vi "test trigger.vi"() -> ()   [LabVIEW 2012]
uses:
  <vilib>/Instr/_visa.llb/VISA Configure Serial Port (Instr).vi
  <vilib>/DAQmx/write.llb/DAQmx Write (Analog 1D Wfm NChan NSamp).vi
  <vilib>/DAQmx/configure/timing.llb/DAQmx Timing (Sample Clock).vi
  <resource>/objmgr/daqmx.rc
  <vilib>/measure/NI_MABase.lvlib
  <vilib>/DAQmx/configure/trigger.llb/DAQmx Start Trigger (Digital Edge).vi
  <vilib>/DAQmx/configure/trigger.llb/DAQmx Start Trigger (Analog Edge).vi
  <vilib>/DAQmx/configure/trigger.llb/DAQmx Reference Trigger (Digital Edge).vi
  <vilib>/DAQmx/configure/trigger.llb/DAQmx Reference Trigger (Analog Edge).vi
  <vilib>/DAQmx/read.llb/DAQmx Read (Analog 1D Wfm NChan NSamp).vi
  <vilib>/DAQmx/configure/task.llb/DAQmx Configure Logging (TDMS).vi
  <vilib>/DAQmx/create/channels.llb/DAQmx Create Channel (AO-Voltage-Basic).vi
  <vilib>/DAQmx/create/channels.llb/DAQmx Create Channel (AI-Voltage-Basic).vi
panel:
  in  "Line Scan":bool
  out "Move X":bool
  in  "Step X":dbl=0.2
  in  "Emergency Stop":bool
  in  "Stop 3":bool
  in  "Home Y":bool
  in  "Home X":bool
  in  "Back":bool
  in  "Front":bool
  in  "Left":bool
  in  "Right":bool
  in  "Save Speed":bool
  in  "Stop Scan":bool
  in  "Cur. Pos Y":dbl=30.0 format="%#.4f"
  in  "Cur. Pos X":dbl=-33.28 format="%#.4f"
  in  "Travel per Pulse (mm)":dbl=0.002
  in  "2 Rate":dbl=0.4
  in  "1 Rate":dbl=0.2
  in  "Step Y":dbl=0.2
  in  "Y-length":dbl=20.0
  in  "X-length":dbl=20.0
  in  "2 Min":dbl=0.4
  in  "1  Max":dbl=6.0
  in  "2 Max":dbl=6.0
  in  "1 Min":dbl=0.4
  in  "Parity":u16(ring) items=["None", "Odd", "Even", "Mark", "Space"]
  in  "stop bits":u16(ring)=10 items=["1.0"=10, "1.5"=15, "2.0"=20]
  in  "Move Distance (mm)":dbl=10.0
  in  "Data bits":u16=8 min=5 max=8 step=1
  in  "Baud Rate":u32=9600
  in  "COM Port":refnum<visa-resource-name>="COM4"
  in  "Scan":bool
  out "Waveform Graph":waveform(dbl)[](graph)=[{"t0"=timestamp(3527210060.2234635 s since 1904-01-01), "dt"=1.9999999999999944e-06, "Y"=array[5000 elements], "attributes"=variant("NI_ChannelName"=variant(string "Dev4/ai1"), "NI_UnitDescription"=variant(string "Volts"))}]
  out "숫자형":i32=2
  in  "Number of Samples 2":i32=5000
  in  "Trigger Type":T1(tab)=enum."Digital Start"
  in  "Edge":i32(ring)=10280 items=["Rising"=10280, "Falling"=10171]
  in  "Digital Trigger Source":tag="/Dev4/PFI1"
  in  "Level (V)":dbl format="%0.2f"
  in  "Hysteresis (V)":dbl
  in  "Slope":i32(ring)=10280 items=["Rising"=10280, "Falling"=10171]
  in  "Analog Trigger Source":string="APFI0"
  in  "Digital Ref Trigger Source":tag
  in  "Edge 2":i32(ring)=10280 items=["Rising"=10280, "Falling"=10171]
  in  "Pre-Trigger Samples":u32
  in  "Analog Ref Trigger Source":string="APFI0"
  in  "Slope 2":i32(ring)=10280 items=["Rising"=10280, "Falling"=10171]
  in  "Level (V) 2":dbl format="%0.2f"
  in  "Pre-Trigger Samples 2":u32
  in  "TDMS File Path":path
  in  "Sample Rate":dbl=500000.0
  in  "Sample Clock Source 2":tag="OnboardClock"
  in  "Terminal Configuration":i32(ring)=10083 items=["default"=-1, "RSE"=10083, "NRSE"=10078, "Differential"=10106, "Pseudodifferential"=12529]
  in  "Max Voltage":dbl=10.0
  in  "Min Voltage":dbl=-10.0
  in  "Physical Channel":tag="Dev4/ai1"
  out "Actual Sample Rate":dbl=500000.0 format="%0.2f"
  in  "Logging Mode":i32(ring)=10231 items=["Off"=10231, "Log and Read"=15842]
  in  "Stop 4":bool
  out "Actual Sample Rate 2":dbl=500000.0 format="%0.2f"
  in  "Physical Channel(s)":tag="Dev4/ao1"
  in  "Min Voltage 2":dbl=-10.0
  in  "Max Voltage 2":dbl=10.0
  in  "Sample Clock Source":tag="OnboardClock"
  in  "Sample Rate 2":dbl=500000.0
  in  "Number of Samples":i32=6000
  in  "Output Array":T2(array[cluster])=[{"Waveform Type"=2, "Amplitude"=5.0, "Frequency"=2000.0}] {"Frequency" format="%0.2p"; "Amplitude" format="%0.2p"; "Waveform Type" items=["Sine Wave", "Triangle Wave", "Square Wave", "Sawtooth Wave"]}
  in  "Duty cycle %":dbl=50.0 format="%#.2f"
  in  "Pulser Trigger Source":tag="/Dev4/PFI1" caption="소스"
  out "Waveform Graph 2":waveform(dbl)[](graph)=[{"t0"=timestamp(0 s since 1904-01-01), "dt"=2e-06, "Y"=array[6000 elements]}]
  # "Motor"
  # "Measure Pulser"
  # "Pulser Out"
  # "To configure and use a start trigger you must have the necessary tab selected above.  Not all hardware supports triggering--refer to your device documentation for more info."
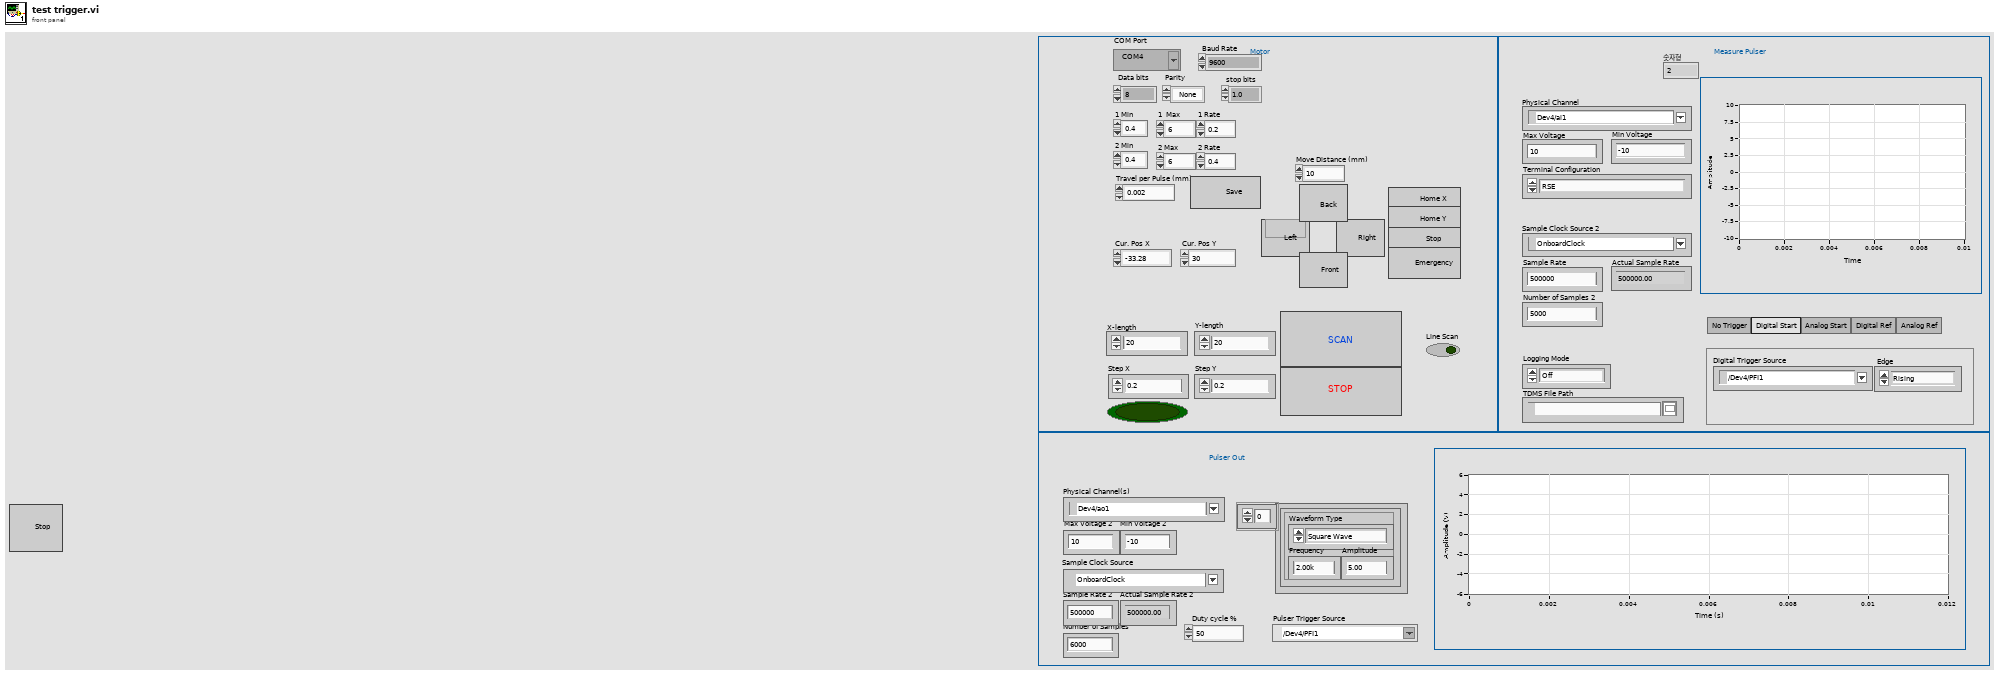
[diagram p1: front panel]
types:
  T1 = enum32{"No Trigger", "Digital Start", "Analog Start", "Digital Ref", "Analog Ref"}
  T2 = cluster{"Waveform Type":u16, "Amplitude":dbl, "Frequency":dbl}[]
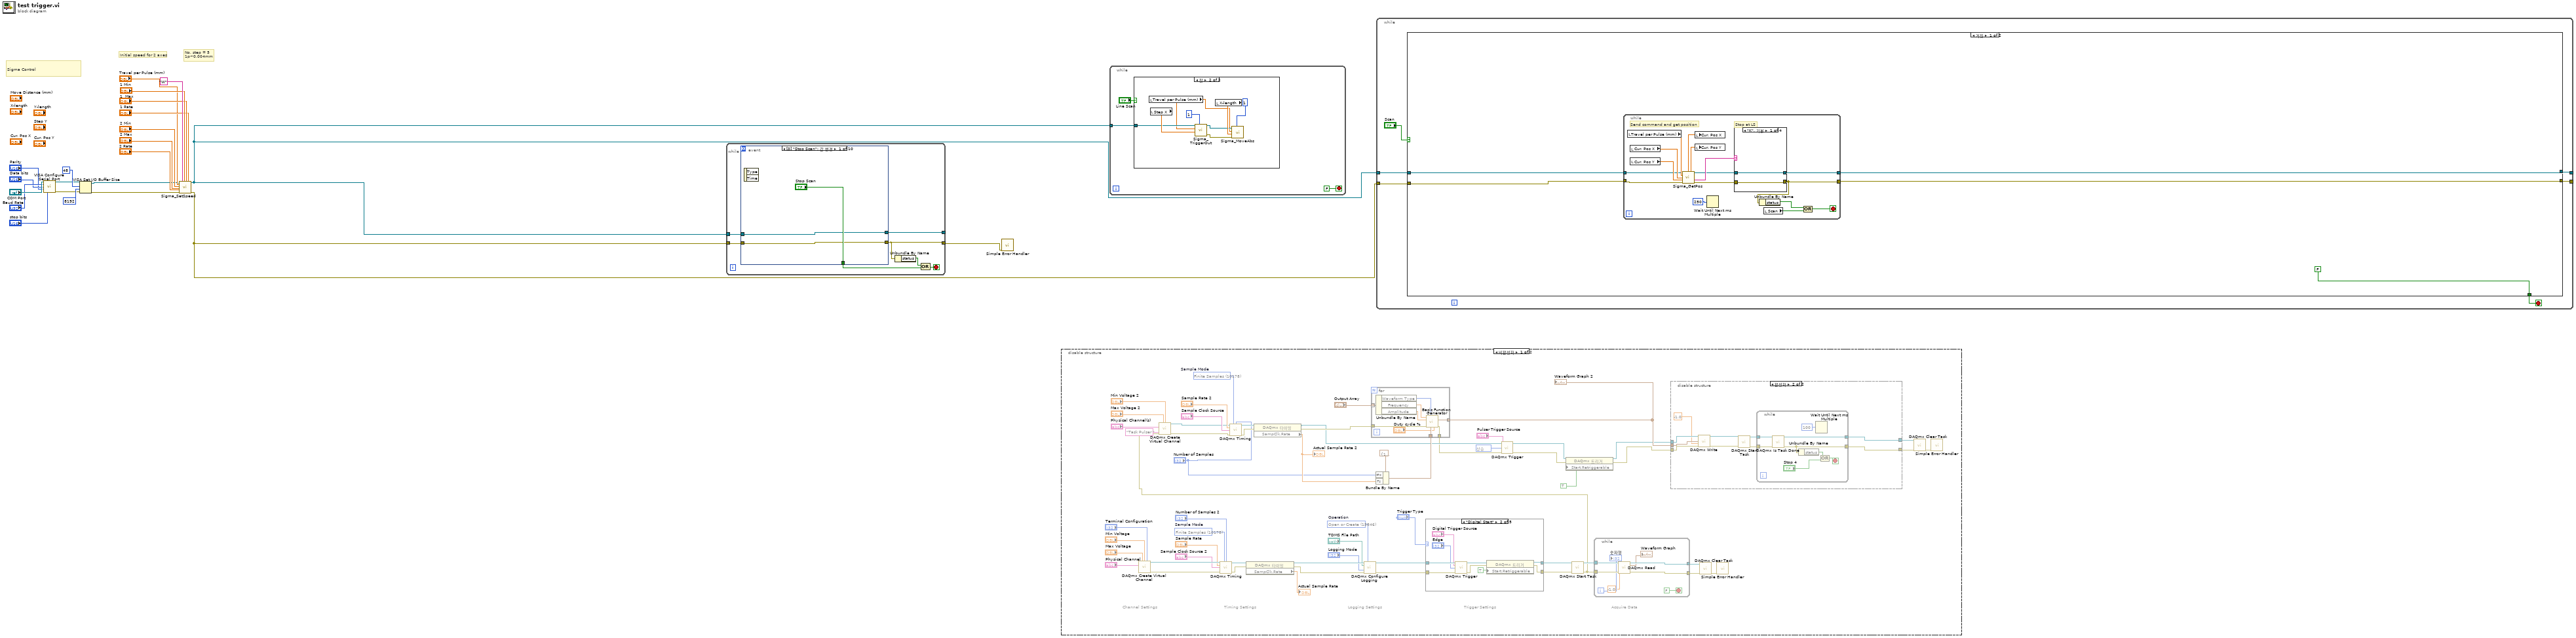
[diagram p0: block diagram]
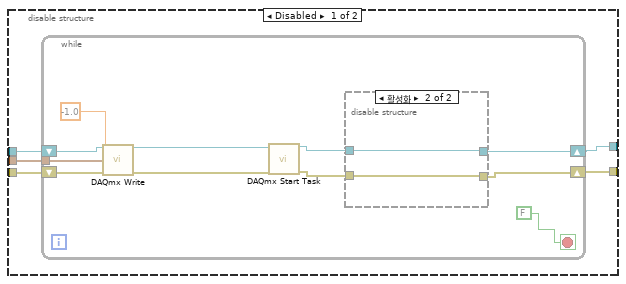
[diagram p2: hidden frame]
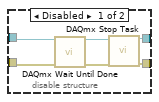
[diagram p3: hidden frame]
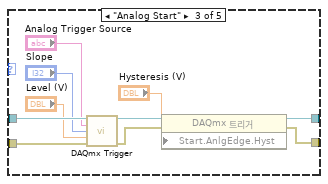
[diagram p5: hidden frame]
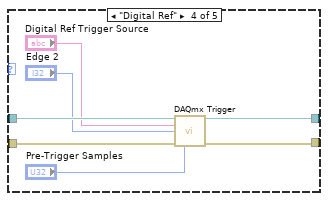
[diagram p6: hidden frame]
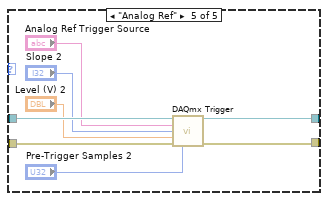
[diagram p7: hidden frame]
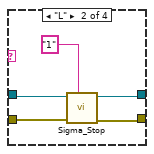
[diagram p10: hidden frame]
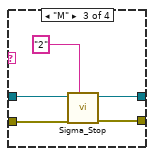
[diagram p11: hidden frame]
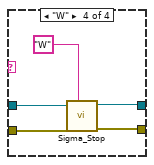
[diagram p12: hidden frame]
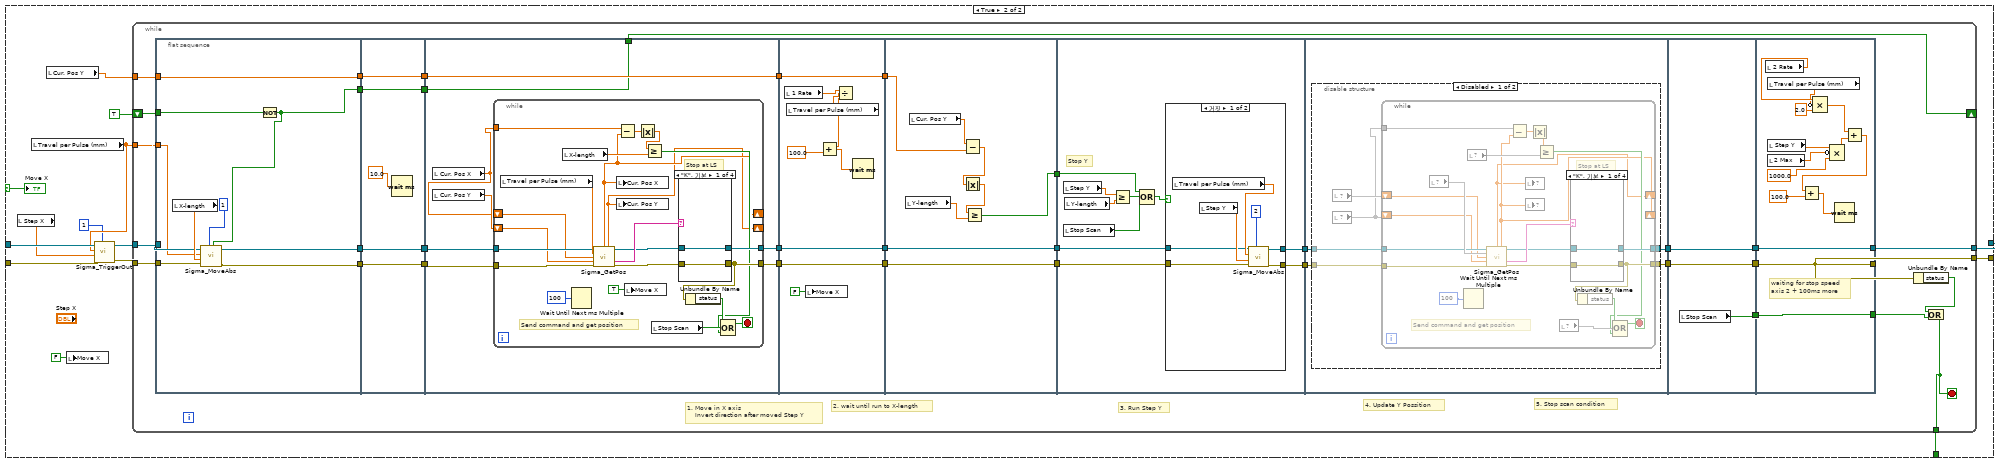
[diagram p13: hidden frame]
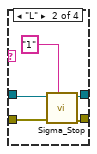
[diagram p14: hidden frame]
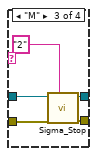
[diagram p15: hidden frame]
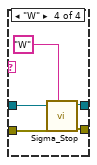
[diagram p16: hidden frame]
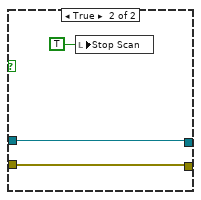
[diagram p17: hidden frame]
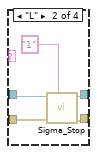
[diagram p18: hidden frame]
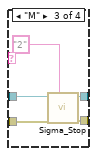
[diagram p19: hidden frame]
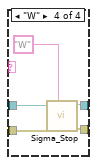
[diagram p20: hidden frame]
diagram:
  # "No. step = 5\n1p~0.004mm"
  # "Initial speed for 2 axes"
  # "Sigma Control"
  n1 = call-poly "VISA Configure Serial Port"("VISA resource name"="COM Port", "baud rate (9600)"="Baud Rate", "data bits (8)"="Data bits", "parity (0:none)"="Parity", "stop bits (10: 1 bit)"="stop bits") -> ("VISA resource name out"=w9:refnum<visa-resource-name>, "error out"=w3:errorcluster)  [unwired: 9 in]
  n2 = VISA Set I/O Buffer Size(VISA resource name=w9, mask (16)=48, size (4096)=u32 8192, error in (no error)=w3) -> (VISA resource name out=w13:refnum<visa-resource-name>, error out=w12:errorcluster)
  n3 = call "Sigma_SetSpeed.vi"("VISA resource name"=w13, "Travel per Pulse (0.004mm)"="Travel per Pulse (mm)", "Min (1mm) 2"="2 Min", "Max (2mm) 2"="2 Max", "Rate (1mm) 2"="2 Rate", "error in (no error)"=w12, "Axis (1)"="W", "Min (1mm)"="1 Min", "Max (2mm)"="1  Max", "Rate (1mm)"="1 Rate") -> ("VISA resource name out"=w1:refnum<visa-resource-name>, "error out"=w2:errorcluster)  [unwired: 8 in]
  n4 = while {
    tunnel: w1 -> [w29]
    tunnel: [w24] -> _
    tunnel: w2 -> [w28]
    tunnel: [w26] -> w22
    stop <- w25 stop-if-true
    n5 = event shown="[0] \"Stop Scan\": 값 변경" {
      selector: _ -> [_ _ _ _ _ _ _ _ _ _]
      dyn-events: _ -> [_ _ _ _ _ _ _ _ _ _]
      timeout: _ -> [_ _ _ _ _ _ _ _ _ _]
      tunnel: w29 -> [w31 w44 w47 w62 w77 w92 w109 w121 w131 w143]
      tunnel: w28 -> [w30 w41 w46 w61 w76 w91 w108 w120 w130 w142]
      tunnel: [w31 w43 w49 w64 w79 w94 w106 w119 w133 w145] -> w24
      tunnel: [w30 w42 w48 w63 w78 w93 w105 w118 w132 w144] -> w26
      tunnel: ["Stop Scan" _ _ _ _ _ _ _ _ _] -> w23
      event "Stop Scan": Value Change {
        n6 = event-data() -> ()  [unwired: 1 in, 2 out]
      }
      event "Save Speed": Value Change {
        n7 = event-data() -> ()  [unwired: 1 in, 5 out]
        n8 = local read "Travel per Pulse (mm)"() -> (w33:dbl)
        n9 = local read "1  Max"() -> (w38:dbl)
        n10 = local read "1 Rate"() -> (w37:dbl)
        n11 = local read "2 Rate"() -> (w34:dbl)
        n12 = local read "2 Max"() -> (w35:dbl)
        n13 = local read "1 Min"() -> (w39:dbl)
        n14 = local read "2 Min"() -> (w36:dbl)
        n15 = call "Sigma_SetSpeed.vi"("VISA resource name"=w44, "Travel per Pulse (0.004mm)"=w33, "Min (1mm) 2"=w36, "Max (2mm) 2"=w35, "Rate (1mm) 2"=w34, "error in (no error)"=w41, "Axis (1)"="W", "Min (1mm)"=w39, "Max (2mm)"=w38, "Rate (1mm)"=w37) -> ("VISA resource name out"=w43:refnum<visa-resource-name>, "error out"=w42:errorcluster)  [unwired: 8 in]
      }
      event "Right": Value Change {
        n16 = event-data() -> ()  [unwired: 1 in, 1 out]
        n17 = case shown="참" "Right" {
          tunnel: [w51 w57] -> w49
          tunnel: [w50 w56] -> w48
          tunnel: w47 -> [w51 w59]
          tunnel: w46 -> [w50 w58]
          frame False {
          }
          frame True {
            n18 = local read "Travel per Pulse (mm)"() -> (w53:dbl)
            n19 = local read "Move Distance (mm)"() -> (w52:dbl)
            n20 = call "Sigma_MoveAbs.vi"("Direction (+)"=FALSE, "Axis (1)"=1, "error in (no error)"=w58, "Travel (1mm)"=w52, "Travel per Pulse (0.004mm)"=w53, "VISA resource name"=w59) -> ("error out"=w56:errorcluster, "VISA resource name out"=w57:refnum<visa-resource-name>)  [unwired: 4 in]
          }
        }
      }
      event "Left": Value Change {
        n21 = event-data() -> ()  [unwired: 1 in, 1 out]
        n22 = case shown="참" "Left" {
          tunnel: [w66 w73] -> w64
          tunnel: [w65 w72] -> w63
          tunnel: w62 -> [w66 w74]
          tunnel: w61 -> [w65 w71]
          frame False {
          }
          frame True {
            n23 = local read "Travel per Pulse (mm)"() -> (w68:dbl)
            n24 = local read "Move Distance (mm)"() -> (w67:dbl)
            n25 = call "Sigma_MoveAbs.vi"("Direction (+)"=TRUE, "Axis (1)"=1, "error in (no error)"=w71, "Travel (1mm)"=w67, "Travel per Pulse (0.004mm)"=w68, "VISA resource name"=w74) -> ("error out"=w72:errorcluster, "VISA resource name out"=w73:refnum<visa-resource-name>)  [unwired: 4 in]
          }
        }
      }
      event "Front": Value Change {
        n26 = event-data() -> ()  [unwired: 1 in, 1 out]
        n27 = case shown="참" "Front" {
          tunnel: [w81 w87] -> w79
          tunnel: [w80 w86] -> w78
          tunnel: w77 -> [w81 w89]
          tunnel: w76 -> [w80 w88]
          frame False {
          }
          frame True {
            n28 = local read "Travel per Pulse (mm)"() -> (w83:dbl)
            n29 = local read "Move Distance (mm)"() -> (w82:dbl)
            n30 = call "Sigma_MoveAbs.vi"("Direction (+)"=FALSE, "Axis (1)"=2, "error in (no error)"=w88, "Travel (1mm)"=w82, "Travel per Pulse (0.004mm)"=w83, "VISA resource name"=w89) -> ("error out"=w86:errorcluster, "VISA resource name out"=w87:refnum<visa-resource-name>)  [unwired: 4 in]
          }
        }
      }
      event "Back": Value Change {
        n31 = event-data() -> ()  [unwired: 1 in, 1 out]
        n32 = case shown="참" "Back" {
          tunnel: [w96 w102] -> w94
          tunnel: [w95 w101] -> w93
          tunnel: w92 -> [w96 w104]
          tunnel: w91 -> [w95 w103]
          frame False {
          }
          frame True {
            n33 = local read "Travel per Pulse (mm)"() -> (w98:dbl)
            n34 = local read "Move Distance (mm)"() -> (w97:dbl)
            n35 = call "Sigma_MoveAbs.vi"("Direction (+)"=TRUE, "Axis (1)"=2, "error in (no error)"=w103, "Travel (1mm)"=w97, "Travel per Pulse (0.004mm)"=w98, "VISA resource name"=w104) -> ("error out"=w101:errorcluster, "VISA resource name out"=w102:refnum<visa-resource-name>)  [unwired: 4 in]
          }
        }
      }
      event "Home X": Value Change {
        n36 = event-data() -> ()  [unwired: 1 in, 1 out]
        n37 = case shown="참" "Home X" {
          tunnel: [w111 w114] -> w106
          tunnel: [w110 w113] -> w105
          tunnel: w109 -> [w111 w116]
          tunnel: w108 -> [w110 w115]
          frame False {
          }
          frame True {
            n38 = call "Sigma_Home.vi"("Axis (1)"="1", "error in (no error)"=w115, "VISA resource name"=w116) -> ("error out"=w113:errorcluster, "VISA resource name out"=w114:refnum<visa-resource-name>)  [unwired: 7 in]
          }
        }
      }
      event "Home Y": Value Change {
        n39 = event-data() -> ()  [unwired: 1 in, 1 out]
        n40 = case shown="참" "Home Y" {
          tunnel: [w123 w126] -> w119
          tunnel: [w122 w125] -> w118
          tunnel: w121 -> [w123 w128]
          tunnel: w120 -> [w122 w127]
          frame False {
          }
          frame True {
            n41 = call "Sigma_Home.vi"("Axis (1)"="2", "error in (no error)"=w127, "VISA resource name"=w128) -> ("error out"=w125:errorcluster, "VISA resource name out"=w126:refnum<visa-resource-name>)  [unwired: 7 in]
          }
        }
      }
      event "Stop 3": Value Change {
        n42 = event-data() -> ()  [unwired: 1 in, 1 out]
        n43 = case shown="참" "Stop 3" {
          tunnel: [w135 w136] -> w133
          tunnel: [w134 w137] -> w132
          tunnel: w131 -> [w135 w139]
          tunnel: w130 -> [w134 w138]
          frame False {
          }
          frame True {
            n44 = call "Sigma_Stop.vi"("Axis (1)"="W", "error in (no error)"=w138, "VISA resource name"=w139) -> ("error out"=w137:errorcluster, "VISA resource name out"=w136:refnum<visa-resource-name>)  [unwired: 7 in]
          }
        }
      }
      event "Emergency Stop": Value Change {
        n45 = event-data() -> ()  [unwired: 1 in, 1 out]
        n46 = case shown="참" "Emergency Stop" {
          tunnel: [w147 w150] -> w145
          tunnel: [w146 w149] -> w144
          tunnel: w143 -> [w147 w152]
          tunnel: w142 -> [w146 w151]
          frame False {
          }
          frame True {
            n47 = call "Sigma_Stop.vi"("Axis (1)"="E", "error in (no error)"=w151, "VISA resource name"=w152) -> ("error out"=w149:errorcluster, "VISA resource name out"=w150:refnum<visa-resource-name>)  [unwired: 7 in]
          }
        }
      }
    }
    n48 = Unbundle By Name(w26) -> ("status"=w27:bool)
    n49 = Compound Arithmetic op=OR(w27, w23) -> (w25:bool)
  }
  n50 = call <vilib>:"Simple Error Handler.vi"("error in (no error)"=w22) -> ()  [unwired: 4 in, 5 out]
  n51 = disable-structure shown="비활성화" {
    frame Disabled {
      w165 = 10280 items=["상승"=10280, "하강"=10171] ("edge")
      w181 = 10178 items=["Finite Samples"=10178, "Continuous Samples"=10123, "Hardware Timed Single Point"=12522]  # Sample Mode
      w203 = 15846 items=["Open"=10437, "Open or Create"=15846, "Create or Replace"=15847, "Create"=15848]  # Operation
      w208 = 10178 items=["Finite Samples"=10178, "Continuous Samples"=10123, "Hardware Timed Single Point"=12522]  # Sample Mode
      # "Acquire Data"
      # "Trigger Settings"
      # "Timing Settings"
      # "Channel Settings"
      # "Logging Settings"
      n52 = call-poly <vilib>:"DAQmx Create Virtual Channel.vi"("maximum value"="Max Voltage", "minimum value"="Min Voltage", "input terminal configuration"="Terminal Configuration", "physical channels"="Physical Channel") -> ("task out"=w206:refnum<k21>, "error out"=w207:errorcluster)  [unwired: 10 in]
      n53 = call-poly <vilib>:"DAQmx Timing.vi"("task/channels in"=w206, "sample mode"=w208, "samples per channel"="Number of Samples 2", "rate"="Sample Rate", "source"="Sample Clock Source 2", "error in"=w207) -> ("task out"=w210:refnum<k21>, "error out"=w209:errorcluster)  [unwired: 8 in]
      n54 = property class="DAQmx 타이밍"(reference=w210, error in=w209) -> (reference out=w205:refnum<k21>, error out=w204:errorcluster, "SampClk.Rate"=→"Actual Sample Rate":dbl)
      n55 = call-poly <vilib>:"DAQmx Configure Logging.vi"("task/channels in"=w205, "operation"=w203, "file path"="TDMS File Path", "logging mode"="Logging Mode", "error in"=w204) -> ("task out"=w202:refnum<k21>, "error out"=w201:errorcluster)  [unwired: 9 in]
      n56 = case shown="\"Digital Start\"" "Trigger Type" {
        tunnel: w202 -> [w271 w280 w290 w297 w305]
        tunnel: w201 -> [w270 w279 w289 w296 w304]
        tunnel: [w271 w275 w287 w295 w299] -> w200
        tunnel: [w270 w274 w286 w294 w300] -> w199
        frame "No Trigger", Default {
        }
        frame "Digital Start" {
          n57 = call-poly <vilib>:"DAQmx Trigger.vi"("task/channels in"=w280, "source"="Digital Trigger Source", "edge"="Edge", "error in"=w279) -> ("task out"=w276:refnum<k21>, "error out"=w273:errorcluster)  [unwired: 10 in]
          n58 = property class="DAQmx 트리거"(reference=w276, error in=w273, "Start.Retriggerable"=TRUE ("시작:추가 옵션:재트리거 가능")) -> (reference out=w275:refnum<k21>, error out=w274:errorcluster)
        }
        frame "Analog Start" {
          n59 = call-poly <vilib>:"DAQmx Trigger.vi"("task/channels in"=w290, "source"="Analog Trigger Source", "slope"="Slope", "level"="Level (V)", "error in"=w289) -> ("task out"=w285:refnum<k21>, "error out"=w284:errorcluster)  [unwired: 9 in]
          n60 = property class="DAQmx 트리거"(reference=w285, error in=w284, "Start.AnlgEdge.Hyst"="Hysteresis (V)") -> (reference out=w287:refnum<k21>, error out=w286:errorcluster)
        }
        frame "Digital Ref" {
          n61 = call-poly <vilib>:"DAQmx Trigger.vi"("task/channels in"=w297, "source"="Digital Ref Trigger Source", "edge"="Edge 2", "error in"=w296, "pretrigger samples per channel"="Pre-Trigger Samples") -> ("task out"=w295:refnum<k21>, "error out"=w294:errorcluster)  [unwired: 9 in]
        }
        frame "Analog Ref" {
          n62 = call-poly <vilib>:"DAQmx Trigger.vi"("task/channels in"=w305, "source"="Analog Ref Trigger Source", "slope"="Slope 2", "level"="Level (V) 2", "error in"=w304, "pretrigger samples per channel"="Pre-Trigger Samples 2") -> ("task out"=w299:refnum<k21>, "error out"=w300:errorcluster)  [unwired: 8 in]
        }
      }
      n63 = call <vilib>:"DAQmx Start Task.vi"("task/channels in"=w200, "error in"=w199) -> ("task out"=w198:refnum<k21>, "error out"=w154:errorcluster)  [unwired: 12 in]
      n64 = call-poly <vilib>:"DAQmx Create Virtual Channel.vi"("maximum value"="Max Voltage 2", "minimum value"="Min Voltage 2", "physical channels"="Physical Channel(s)", "name to assign"="Task Pulser ", "error in"=w154) -> ("task out"=w163:refnum<k21>, "error out"=w162:errorcluster)  [unwired: 9 in]
      n65 = call-poly <vilib>:"DAQmx Timing.vi"("task/channels in"=w163, "sample mode"=w181, "samples per channel"="Number of Samples", "rate"="Sample Rate 2", "source"="Sample Clock Source", "error in"=w162) -> ("task out"=w183:refnum<k21>, "error out"=w182:errorcluster)  [unwired: 8 in]
      n66 = property class="DAQmx 타이밍"(reference=w183, error in=w182) -> (reference out=w168:refnum<k21>, error out=w174:errorcluster, "SampClk.Rate"=w172:dbl)
      "Actual Sample Rate 2" <- w172
      n67 = Bundle By Name(cluster=cluster{"Fs":dbl, "#s":dbl} {"Fs"=1000.0, "#s"=1000.0} ("sampling info"), "#s"="Number of Samples", "Fs"=w172) -> (w171:cluster{"Fs":dbl, "#s":dbl})
      n68 = for {
        tunnel: w174 -> [w219]
        tunnel: w171 -> [w218]
        tunnel: [w217] -> w167
        tunnel: "Output Array" -> [w216] mode=indexing
        tunnel: [w213] -> w170 mode=indexing
        n69 = Unbundle By Name(w216) -> ("Waveform Type"=w215:u16, "Frequency"=w214:dbl, "Amplitude"=w211:dbl)
        n70 = call <vilib>:"Basic Function Generator.vi"("square wave duty cycle (%)"="Duty cycle %", "sampling info"=w218, "signal type"=w215, "error in (no error)"=w219, "amplitude"=w211, "frequency"=w214) -> ("error out"=w217:errorcluster, "signal out"=w213:waveform(dbl))  [unwired: 3 in, 1 out]
      }
      "Waveform Graph 2" <- w170
      n71 = call-poly <vilib>:"DAQmx Trigger.vi"("task/channels in"=w168, "source"="Pulser Trigger Source", "edge"=w165, "error in"=w167) -> ("task out"=w159:refnum<k21>, "error out"=w155:errorcluster)  [unwired: 10 in]
      n72 = property class="DAQmx 트리거"(reference=w159, error in=w155, "Start.Retriggerable"=TRUE) -> (reference out=w158:refnum<k21>, error out=w157:errorcluster)
      n73 = while {
        tunnel: w198 -> [w269]
        tunnel: w154 -> [w268]
        tunnel: [w267] -> w197
        tunnel: [w266] -> w196
        i -> [w264]
        stop <- FALSE stop-if-true
        n74 = call-poly <vilib>:"DAQmx Read.vi"("task/channels in"=w269, "timeout"=-1.0, "error in"=w268) -> ("task out"=w267:refnum<k21>, "data"=→"Waveform Graph":waveform(dbl)[], "error out"=w266:errorcluster)  [unwired: 10 in]
        "숫자형" <- w264
      }
      n75 = disable-structure shown="활성화" {
        disable-tunnel: w170 -> [w224 w247]
        disable-tunnel: [w223 w246] -> w161
        disable-tunnel: [w222 w245] -> w160
        disable-tunnel: w158 -> [w221 w249]
        disable-tunnel: w157 -> [w220 w248]
        frame Disabled {
          n76 = while {
            tunnel: w224 -> [w235]
            shift-right: [w231] -> w223
            shift-left: w221 -> [w229]
            shift-right: [w230] -> w222
            shift-left: w220 -> [w228]
            stop <- FALSE stop-if-true
            n77 = call-poly <vilib>:"DAQmx Write.vi"("task/channels in"=w229, "data"=w235, "timeout"=-1.0, "error in"=w228) -> ("task out"=w234:refnum<k21>, "error out"=w233:errorcluster)  [unwired: 9 in, 1 out]
            n78 = call <vilib>:"DAQmx Start Task.vi"("task/channels in"=w234, "error in"=w233) -> ("task out"=w227:refnum<k21>, "error out"=w226:errorcluster)  [unwired: 12 in]
            n79 = disable-structure shown="활성화" {
              disable-tunnel: [w241 w243] -> w231
              disable-tunnel: [w240 w242] -> w230
              disable-tunnel: w227 -> [w239 w243]
              disable-tunnel: w226 -> [w238 w242]
              frame Disabled {
                n80 = call <vilib>:"DAQmx Wait Until Done.vi"("task/channels in"=w239, "error in"=w238) -> ("task out"=w237:refnum<k21>, "error out"=w236:errorcluster)  [unwired: 12 in]
                n81 = call <vilib>:"DAQmx Stop Task.vi"("task/channels in"=w237, "error in"=w236) -> ("task out"=w241:refnum<k21>, "error out"=w240:errorcluster)  [unwired: 12 in]
              }
              frame Enabled {
              }
            }
          }
        }
        frame Enabled {
          n82 = call-poly <vilib>:"DAQmx Write.vi"("task/channels in"=w249, "data"=w247, "timeout"=-1.0, "error in"=w248) -> ("task out"=w251:refnum<k21>, "error out"=w253:errorcluster)  [unwired: 9 in, 1 out]
          n83 = call <vilib>:"DAQmx Start Task.vi"("task/channels in"=w251, "error in"=w253) -> ("task out"=w250:refnum<k21>, "error out"=w252:errorcluster)  [unwired: 12 in]
          n84 = while {
            tunnel: w250 -> [w261]
            tunnel: w252 -> [w260]
            tunnel: [w258] -> w245
            tunnel: [w259] -> w246
            stop <- w254 stop-if-true
            n85 = call <vilib>:"DAQmx Is Task Done.vi"("task/channels in"=w261, "error in"=w260) -> ("task out"=w259:refnum<k21>, "error out"=w258:errorcluster)  [unwired: 11 in, 1 out]
            n86 = Unbundle By Name(w258) -> ("status"=w255:bool)
            n87 = Wait Until Next ms Multiple(millisecond multiple=u32 100) -> ()  [unwired: 1 out]
            n88 = Compound Arithmetic op=OR(w255, "Stop 4") -> (w254:bool)
          }
        }
      }
      n89 = call <vilib>:"DAQmx Clear Task.vi"("task in"=w197, "error in"=w196) -> ("error out"=w195:errorcluster)  [unwired: 13 in]
      n90 = call <vilib>:"Simple Error Handler.vi"("error in (no error)"=w195) -> ()  [unwired: 4 in, 5 out]
      n91 = call <vilib>:"DAQmx Clear Task.vi"("task in"=w161, "error in"=w160) -> ("error out"=w180:errorcluster)  [unwired: 13 in]
      n92 = call <vilib>:"Simple Error Handler.vi"("error in (no error)"=w180) -> ()  [unwired: 4 in, 5 out]
    }
    frame Enabled {
    }
  }
  n93 = while {
    tunnel: w1 -> [w308]
    stop <- FALSE stop-if-true
    n94 = case shown="참" "Line Scan" {
      tunnel: w308 -> [_ w310]
      frame False {
      }
      frame True {
        n95 = local read "Travel per Pulse (mm)"() -> (w309:dbl)
        n96 = local read "Step X"() -> (w315:dbl)
        n97 = call "Sigma_TriggerOut.vi"("Axis(1)"=1, "Trigger distance (mm)"=w315, "Travel per Pulse (mm)"=w309, "VISA resource name"=w310) -> ("error out"=w311:errorcluster, "VISA resource name out"=w312:refnum<visa-resource-name>)  [unwired: 6 in]
        n98 = local read "X-length"() -> (w313:dbl)
        n99 = call "Sigma_MoveAbs.vi"("Axis (1)"=1, "error in (no error)"=w311, "Travel (1mm)"=w313, "Travel per Pulse (0.004mm)"=w309, "VISA resource name"=w312) -> ()  [unwired: 5 in, 2 out]
      }
    }
  }
  n100 = while {
    tunnel: w1 -> [w322]
    tunnel: [w320] -> _
    tunnel: w2 -> [w321]
    tunnel: [w319] -> _
    stop <- w318 stop-if-true
    n101 = case shown="거짓" "Scan" {
      selector: "Scan" -> [_ w369]
      tunnel: [w324 w371] -> w320
      tunnel: w322 -> [w326 w368]
      tunnel: w321 -> [w325 w365]
      tunnel: [w323 w370] -> w319
      tunnel: [FALSE w373] -> w318
      frame False {
        n102 = while {
          tunnel: w325 -> [w335]
          tunnel: [w330] -> w324
          tunnel: [w329] -> w323
          tunnel: w326 -> [w328]
          stop <- w342 stop-if-true
          # "Stop at LS"
          # "Send command and get position"
          n103 = local read "Travel per Pulse (mm)"() -> (w338:dbl)
          n104 = local read "Cur. Pos X"() -> (w332:dbl)
          n105 = local read "Cur. Pos Y"() -> (w331:dbl)
          n106 = call "Sigma_GetPos.vi"("VISA resource name"=w328, "Travel per Pulse (mm)"=w338, "Init Pos X (mm)"=w332, "Init  Pos Y (mm)"=w331, "error in (no error)"=w335) -> ("Pos X (mm)"=w334:dbl, "Pos Y (mm)"=w333:dbl, "VISA resource name out"=w337:refnum<visa-resource-name>, "State String"=w339:string, "error out"=w336:errorcluster)  [unwired: 6 in]
          n107 = local write "Cur. Pos X"(w334) -> ()
          n108 = local write "Cur. Pos Y"(w333) -> ()
          n109 = Wait Until Next ms Multiple(millisecond multiple=u32 250) -> ()  [unwired: 1 out]
          n110 = case shown="\"K\", 기본" w339 {
            tunnel: [w345 w350 w355 w360] -> w330
            tunnel: [w344 w349 w354 w359] -> w329
            tunnel: w337 -> [w345 w347 w352 w357]
            tunnel: w336 -> [w344 w346 w351 w356]
            frame "K", Default {
            }
            frame "L" {
              n111 = call "Sigma_Stop.vi"("Axis (1)"="1", "error in (no error)"=w346, "VISA resource name"=w347) -> ("error out"=w349:errorcluster, "VISA resource name out"=w350:refnum<visa-resource-name>)  [unwired: 7 in]
            }
            frame "M" {
              n112 = call "Sigma_Stop.vi"("Axis (1)"="2", "error in (no error)"=w351, "VISA resource name"=w352) -> ("error out"=w354:errorcluster, "VISA resource name out"=w355:refnum<visa-resource-name>)  [unwired: 7 in]
            }
            frame "W" {
              n113 = call "Sigma_Stop.vi"("Axis (1)"="W", "error in (no error)"=w356, "VISA resource name"=w357) -> ("error out"=w359:errorcluster, "VISA resource name out"=w360:refnum<visa-resource-name>)  [unwired: 7 in]
            }
          }
          n114 = Unbundle By Name(w329) -> ("status"=w343:bool)
          n115 = local read "Scan"() -> (w341:bool)
          n116 = Compound Arithmetic op=OR(w343, w341) -> (w342:bool)
        }
      }
      frame True {
        n117 = local read "Step X"() -> (w364:dbl)
        n118 = local read "Travel per Pulse (mm)"() -> (w363:dbl)
        n119 = local read "Cur. Pos Y"() -> (w374:dbl)
        n120 = local write "Move X"(FALSE ("Move X")) -> ()
        n121 = call "Sigma_TriggerOut.vi"("Axis(1)"=1, "error in (no error)"=w365, "Trigger distance (mm)"=w364, "Travel per Pulse (mm)"=w363, "VISA resource name"=w368) -> ("error out"=w366:errorcluster, "VISA resource name out"=w367:refnum<visa-resource-name>)  [unwired: 5 in]
        n122 = while {
          shift-right: [w394] -> _
          shift-left: TRUE ("Direction (+)") -> [w407]
          tunnel: w374 -> [w406]
          tunnel: [w402] -> w373
          tunnel: w367 -> [w409]
          tunnel: w366 -> [w408]
          tunnel: [w395] -> w371
          tunnel: [w392] -> w370
          tunnel: w363 -> [w383]
          stop <- w402 stop-if-true
          # "5. Stop scan condition"
          # "3. Run Step Y"
          # "2. wait until run to X-length"
          # "1. Move in X axis\n    Invert direction after moved Step Y"
          # "4. Update Y Possition"
          n123 = flat-sequence {
            tunnel: w409 -> [w414]
            tunnel: w408 -> [w413]
            tunnel: w407 -> [w419]
            tunnel: w406 -> [w417]
            tunnel: [w418] -> w382
            tunnel: [w412] -> w380
            tunnel: [w411] -> w378
            tunnel: [w417] -> w376
            tunnel: w383 -> [w410]
            tunnel: w382 -> [w424]
            tunnel: [w424] -> w381
            tunnel: w380 -> [w423]
            tunnel: [w423] -> w379
            tunnel: w378 -> [w422]
            tunnel: [w422] -> w377
            tunnel: w376 -> [w421]
            tunnel: [w421] -> w375
            tunnel: w381 -> [w427]
            tunnel: w379 -> [w432]
            tunnel: w377 -> [w431]
            tunnel: w375 -> [w428]
            tunnel: [w430] -> w401
            tunnel: [w429] -> w400
            tunnel: [w428] -> w396
            tunnel: [w427] -> w394
            tunnel: [w480] -> w391
            tunnel: w401 -> [w480]
            tunnel: [w479] -> w389
            tunnel: w400 -> [w479]
            tunnel: [w478] -> w387
            tunnel: w396 -> [w478]
            tunnel: w391 -> [w488]
            tunnel: [w488] -> w390
            tunnel: w389 -> [w487]
            tunnel: [w487] -> w388
            tunnel: w387 -> [w482]
            tunnel: [w483] -> w386
            tunnel: [w498] -> w405
            tunnel: [w497] -> w404
            tunnel: w390 -> [w494]
            tunnel: w388 -> [w493]
            tunnel: w386 -> [w490]
            tunnel: w405 -> [w512]
            tunnel: w404 -> [w511]
            tunnel: [w510] -> w397
            tunnel: [w509] -> w393
            tunnel: [w561] -> w399
            tunnel: [w560] -> w398
            tunnel: w397 -> [w560]
            tunnel: w393 -> [w561]
            tunnel: [w559] -> w384
            tunnel: w399 -> [w574]
            tunnel: [w575] -> w392
            tunnel: w398 -> [w575]
            tunnel: [w574] -> w395
            tunnel: [w573] -> w385
            tunnel: w384 -> [w573]
            frame #0 {
              n124 = local read "X-length"() -> (w416:dbl)
              n125 = Not(x=w419) -> (.not. x?=w418:bool)
              n126 = call "Sigma_MoveAbs.vi"("Direction (+)"=w418, "Axis (1)"=1, "error in (no error)"=w413, "Travel (1mm)"=w416, "Travel per Pulse (0.004mm)"=w410, "VISA resource name"=w414) -> ("error out"=w411:errorcluster, "VISA resource name out"=w412:refnum<visa-resource-name>)  [unwired: 4 in]
            }
            frame #1 {
              n127 = Wait (ms)(milliseconds to wait=10.0 ("y")) -> ()  [unwired: 1 out]
            }
            frame #2 {
              n128 = local read "Cur. Pos X"() -> (w425:dbl)
              n129 = local read "Cur. Pos Y"() -> (w426:dbl)
              n130 = while {
                tunnel: w432 -> [w445]
                tunnel: w431 -> [w446]
                tunnel: [w444] -> w430
                tunnel: [w443] -> w429
                shift-right: [w437] -> _
                shift-left: w426 -> [w436]
                shift-right: [w438] -> _
                shift-left: w425 -> [w435]
                tunnel: w425 -> [w434]
                stop <- w453 stop-if-true
                # "Stop at LS"
                # "Send command and get position"
                n131 = local read "Travel per Pulse (mm)"() -> (w449:dbl)
                n132 = local read "X-length"() -> (w441:dbl)
                n133 = Wait Until Next ms Multiple(millisecond multiple=u32 100) -> ()  [unwired: 1 out]
                n134 = call "Sigma_GetPos.vi"("VISA resource name"=w445, "Travel per Pulse (mm)"=w449, "Init Pos X (mm)"=w435, "Init  Pos Y (mm)"=w436, "error in (no error)"=w446) -> ("Pos X (mm)"=w438:dbl, "Pos Y (mm)"=w437:dbl, "VISA resource name out"=w448:refnum<visa-resource-name>, "State String"=w450:string, "error out"=w447:errorcluster)  [unwired: 6 in]
                n135 = local write "Cur. Pos X"(w438) -> ()
                n136 = local write "Cur. Pos Y"(w437) -> ()
                n137 = Subtract(x=w434, y=w438) -> (x-y=w440:dbl)
                n138 = local write "Move X"(TRUE ("Move X")) -> ()
                n139 = Absolute Value(x=w440) -> (abs(x)=w442:dbl)
                n140 = Greater Or Equal?(x=w442, y=w441) -> (x >= y?=w439:bool)
                n141 = local read "Stop Scan"() -> (w452:bool)
                n142 = case shown="\"K\", 기본" w450 {
                  tunnel: [w456 w461 w466 w471] -> w444
                  tunnel: [w455 w460 w465 w470] -> w443
                  tunnel: w448 -> [w456 w458 w463 w468]
                  tunnel: w447 -> [w455 w457 w462 w467]
                  frame "K", Default {
                  }
                  frame "L" {
                    n143 = call "Sigma_Stop.vi"("Axis (1)"="1", "error in (no error)"=w457, "VISA resource name"=w458) -> ("error out"=w460:errorcluster, "VISA resource name out"=w461:refnum<visa-resource-name>)  [unwired: 7 in]
                  }
                  frame "M" {
                    n144 = call "Sigma_Stop.vi"("Axis (1)"="2", "error in (no error)"=w462, "VISA resource name"=w463) -> ("error out"=w465:errorcluster, "VISA resource name out"=w466:refnum<visa-resource-name>)  [unwired: 7 in]
                  }
                  frame "W" {
                    n145 = call "Sigma_Stop.vi"("Axis (1)"="W", "error in (no error)"=w467, "VISA resource name"=w468) -> ("error out"=w470:errorcluster, "VISA resource name out"=w471:refnum<visa-resource-name>)  [unwired: 7 in]
                  }
                }
                n146 = Unbundle By Name(w443) -> ("status"=w454:bool)
                n147 = Compound Arithmetic op=OR(w454, w452, w439) -> (w453:bool)
              }
            }
            frame #3 {
              n148 = local read "1 Rate"() -> (w476:dbl)
              n149 = local read "Travel per Pulse (mm)"() -> (w477:dbl)
              n150 = local write "Move X"(FALSE ("Move X")) -> ()
              n151 = Divide(x=w476, y=w477) -> (x/y=w473:dbl)
              n152 = Add(x=w473, y=100.0) -> (x+y=w475:dbl)
              n153 = Wait (ms)(milliseconds to wait=w475) -> ()  [unwired: 1 out]
            }
            frame #4 {
              n154 = local read "Y-length"() -> (w481:dbl)
              n155 = local read "Cur. Pos Y"() -> (w486:dbl)
              n156 = Subtract(x=w486, y=w482) -> (x-y=w485:dbl)
              n157 = Absolute Value(x=w485) -> (abs(x)=w484:dbl)
              n158 = Greater Or Equal?(x=w484, y=w481) -> (x >= y?=w483:bool)
            }
            frame #5 {
              # "Stop Y"
              n159 = local read "Step Y"() -> (w496:dbl)
              n160 = local read "Stop Scan"() -> (w492:bool)
              n161 = local read "Y-length"() -> (w495:dbl)
              n162 = Greater Or Equal?(x=w496, y=w495) -> (x >= y?=w491:bool)
              n163 = Compound Arithmetic op=OR(w490, w491, w492) -> (w489:bool)
              n164 = case shown="거짓" w489 {
                tunnel: [w503 w508] -> w498
                tunnel: [w502 w507] -> w497
                tunnel: w494 -> [w500 w508]
                tunnel: w493 -> [w499 w507]
                frame False {
                  n165 = local read "Travel per Pulse (mm)"() -> (w501:dbl)
                  n166 = local read "Step Y"() -> (w505:dbl)
                  n167 = call "Sigma_MoveAbs.vi"("Axis (1)"=2, "error in (no error)"=w499, "Travel (1mm)"=w505, "Travel per Pulse (0.004mm)"=w501, "VISA resource name"=w500) -> ("error out"=w502:errorcluster, "VISA resource name out"=w503:refnum<visa-resource-name>)  [unwired: 5 in]
                }
                frame True {
                  n168 = local write "Stop Scan"(TRUE ("Stop Scan")) -> ()
                }
              }
            }
            frame #6 {
              n169 = disable-structure shown="Disabled" {
                disable-tunnel: w512 -> [w518 w558]
                disable-tunnel: w511 -> [w517 w557]
                disable-tunnel: [w516 w557] -> w510
                disable-tunnel: [w515 w558] -> w509
                frame Disabled {
                  n170 = local read item#-1() -> (w514)
                  n171 = local read item#-1() -> (w513)
                  n172 = while {
                    tunnel: w518 -> [w530]
                    tunnel: w517 -> [w531]
                    tunnel: [w529] -> w515
                    tunnel: [w528] -> w516
                    shift-right: [w523] -> _
                    shift-left: w513 -> [w520]
                    shift-right: [w522] -> _
                    shift-left: w514 -> [w521]
                    tunnel: w513 -> [w519]
                    stop <- w538 stop-if-true
                    # "Stop at LS"
                    # "Send command and get position"
                    n173 = local read item#-1() -> (w534)
                    n174 = Wait Until Next ms Multiple(millisecond multiple=u32 100) -> ()  [unwired: 1 out]
                    n175 = local read item#-1() -> (w526)
                    n176 = call "Sigma_GetPos.vi"("VISA resource name"=w530, "Travel per Pulse (mm)"=w534, "Init Pos X (mm)"=w521, "Init  Pos Y (mm)"=w520, "error in (no error)"=w531) -> ("Pos X (mm)"=w522:dbl, "Pos Y (mm)"=w523:dbl, "VISA resource name out"=w533:refnum<visa-resource-name>, "State String"=w535:string, "error out"=w532:errorcluster)  [unwired: 6 in]
                    n177 = Subtract(x=w519, y=w523) -> (x-y=w525:dbl)
                    n178 = local write item#-1(w522) -> ()
                    n179 = local write item#-1(w523) -> ()
                    n180 = Absolute Value(x=w525) -> (abs(x)=w527:dbl)
                    n181 = Greater Or Equal?(x=w527, y=w526) -> (x >= y?=w524:bool)
                    n182 = local read item#-1() -> (w537)
                    n183 = case shown="\"K\", 기본" w535 {
                      tunnel: [w541 w546 w551 w556] -> w529
                      tunnel: [w540 w545 w550 w555] -> w528
                      tunnel: w533 -> [w541 w543 w548 w553]
                      tunnel: w532 -> [w540 w542 w547 w552]
                      frame "K", Default {
                      }
                      frame "L" {
                        n184 = call "Sigma_Stop.vi"("Axis (1)"="1", "error in (no error)"=w542, "VISA resource name"=w543) -> ("error out"=w545:errorcluster, "VISA resource name out"=w546:refnum<visa-resource-name>)  [unwired: 7 in]
                      }
                      frame "M" {
                        n185 = call "Sigma_Stop.vi"("Axis (1)"="2", "error in (no error)"=w547, "VISA resource name"=w548) -> ("error out"=w550:errorcluster, "VISA resource name out"=w551:refnum<visa-resource-name>)  [unwired: 7 in]
                      }
                      frame "W" {
                        n186 = call "Sigma_Stop.vi"("Axis (1)"="W", "error in (no error)"=w552, "VISA resource name"=w553) -> ("error out"=w555:errorcluster, "VISA resource name out"=w556:refnum<visa-resource-name>)  [unwired: 7 in]
                      }
                    }
                    n187 = Unbundle By Name(w528) -> ("status"=w539:bool)
                    n188 = Compound Arithmetic op=OR(w539, w537, w524) -> (w538:bool)
                  }
                }
                frame Enabled {
                }
              }
            }
            frame #7 {
              n189 = local read "Stop Scan"() -> (w559:bool)
            }
            frame #8 {
              # "waiting for stop speed\naxis 2 + 100ms more"
              n190 = local read "2 Rate"() -> (w565:dbl)
              n191 = local read "Travel per Pulse (mm)"() -> (w564:dbl)
              n192 = local read "2 Max"() -> (w571:dbl)
              n193 = local read "Step Y"() -> (w572:dbl)
              n194 = Compound Arithmetic op=MULTIPLY(w565, invert w564, 2.0 ("value")) -> (w562:dbl)
              n195 = Compound Arithmetic op=MULTIPLY(w572, invert w571, 1000.0 ("value")) -> (w569:dbl)
              n196 = Add(x=w562, y=w569) -> (x+y=w568:dbl)
              n197 = Add(x=w568, y=100.0) -> (x+y=w566:dbl)
              n198 = Wait (ms)(milliseconds to wait=w566) -> ()  [unwired: 1 out]
            }
          }
          n199 = Unbundle By Name(w392) -> ("status"=w403:bool)
          n200 = Compound Arithmetic op=OR(w403, w385) -> (w402:bool)
        }
        "Move X" <- w369
      }
    }
  }
